vi "quiz3.vi"() -> ()   [LabVIEW 2017]
panel:
  out "Tab Control":enum32{"Login", "Menu", "Add", "delete"}(tab)
  in  "Ingresar":bool
  in  "Contraseña":string
  in  "Usuario":string
  in  "Delete Button":bool
  in  "Add Button":bool
  in  "Home Button":bool
  out "Cusuario":string
  in  "Previous Button":bool
  in  "AddContraseña":string
  in  "AddUsuario":string
  in  "Agregar":bool
  out "Agregado":bool
  in  "Cancel Button":bool
  in  "DeleteUsuario 2":string
  in  "Previous Button 2":bool
  out "text":string
  # "USTED INGRESO CON EL USUARIO"
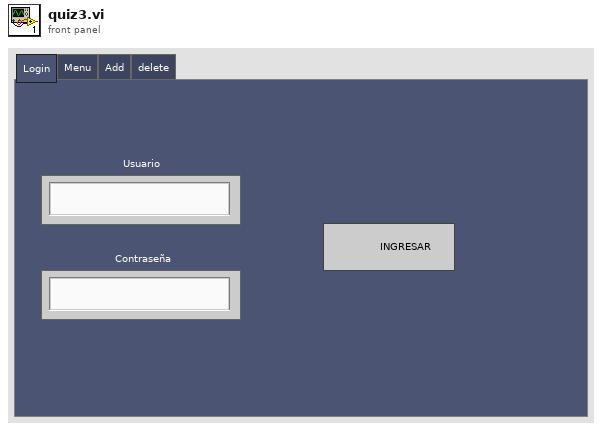
[diagram p1: front panel]
types:
  T1 = enum16{"open", "replace", "create", "open or create", "replace or create", "replace or create with confirmation"}
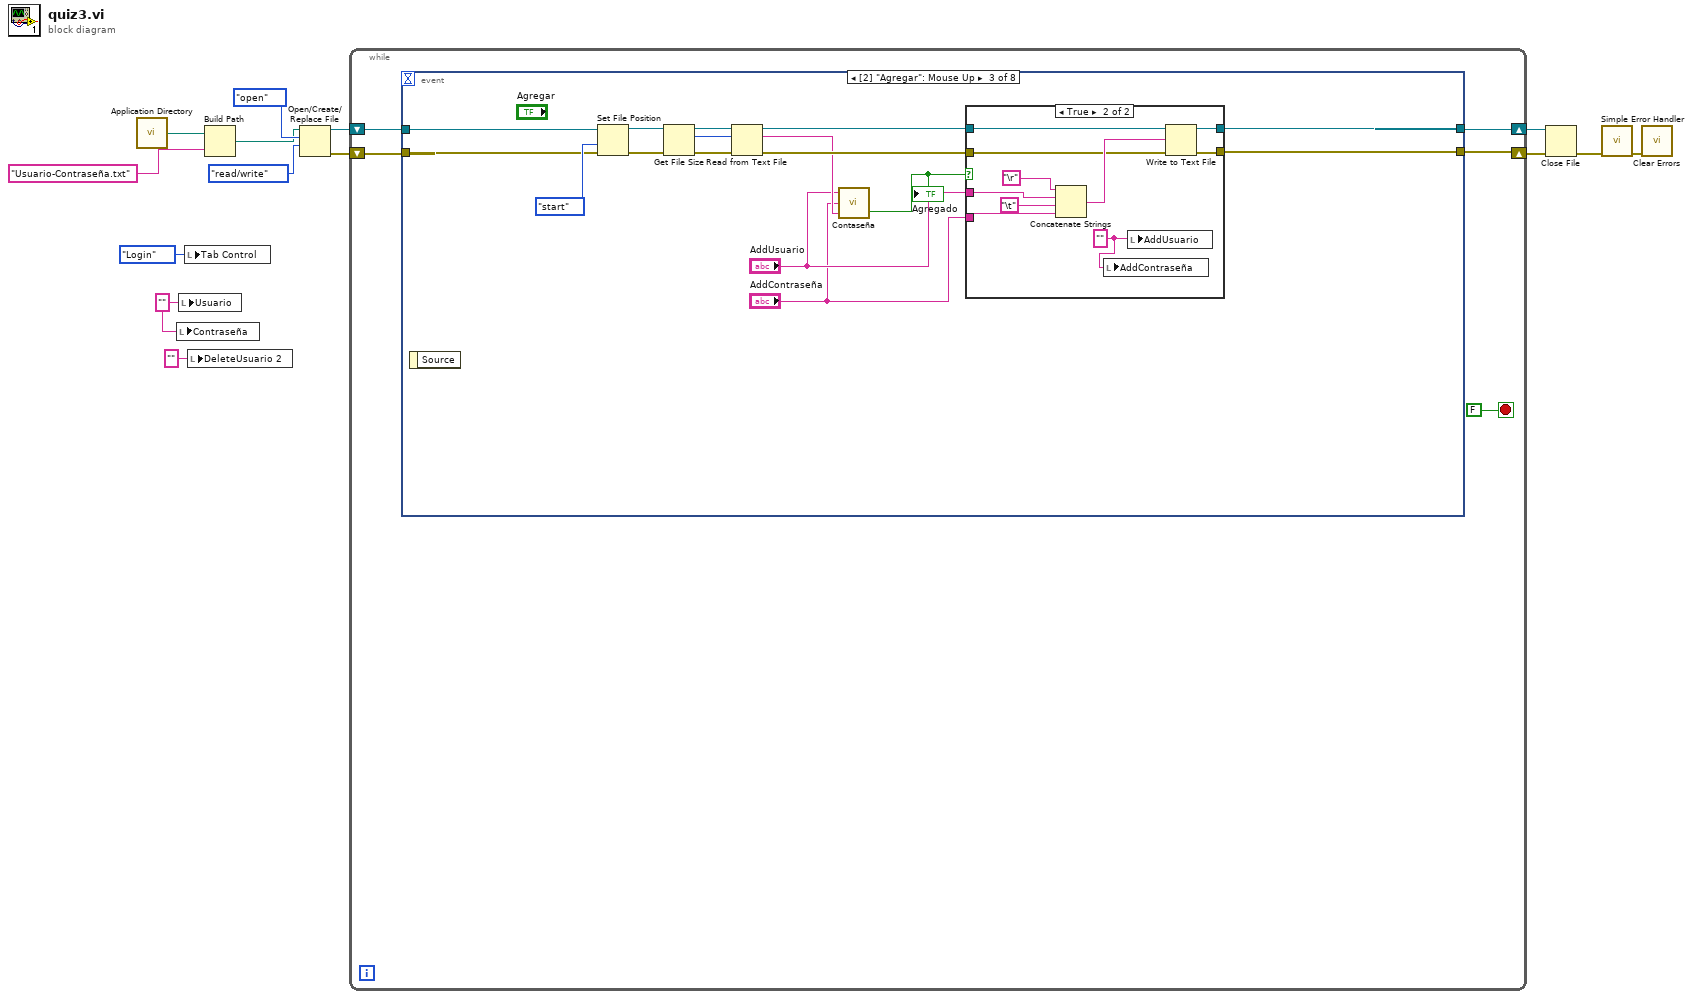
[diagram p0: block diagram]
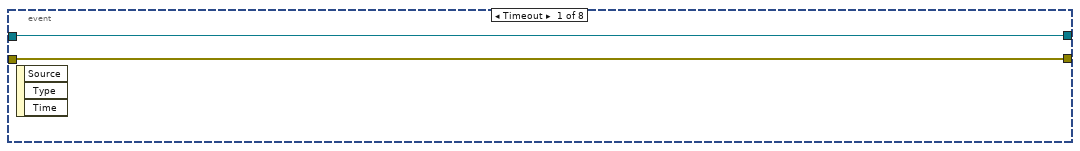
[diagram p2: hidden frame]
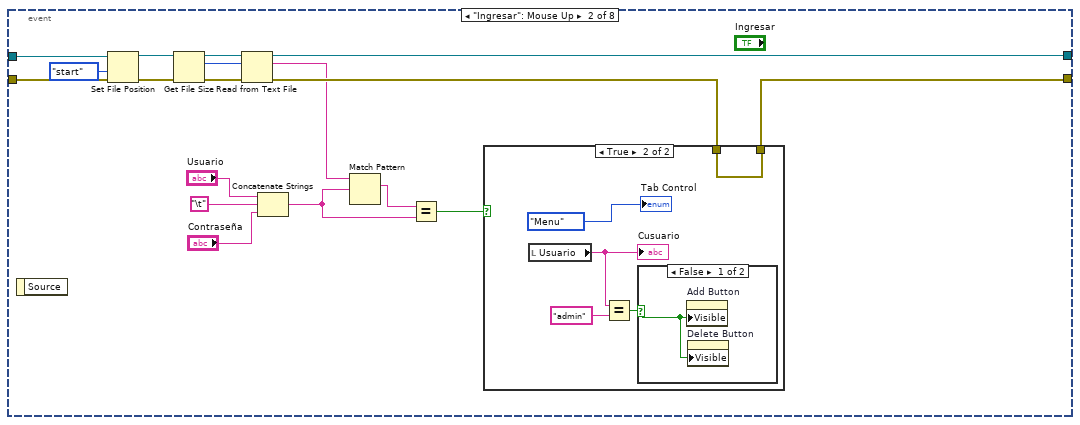
[diagram p3: hidden frame]
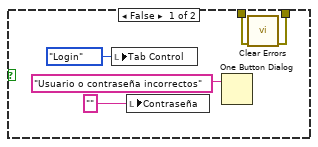
[diagram p4: hidden frame]
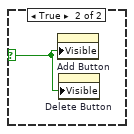
[diagram p5: hidden frame]
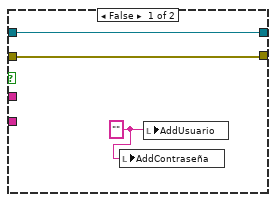
[diagram p6: hidden frame]
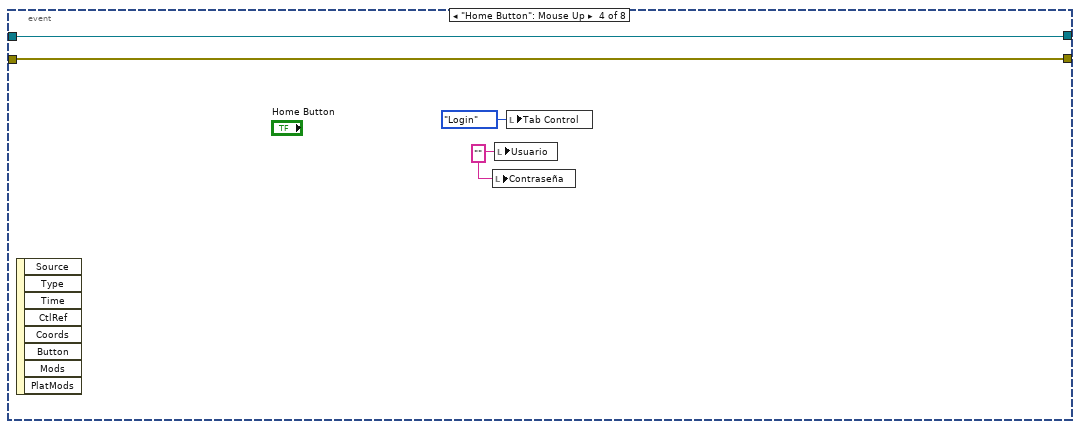
[diagram p7: hidden frame]
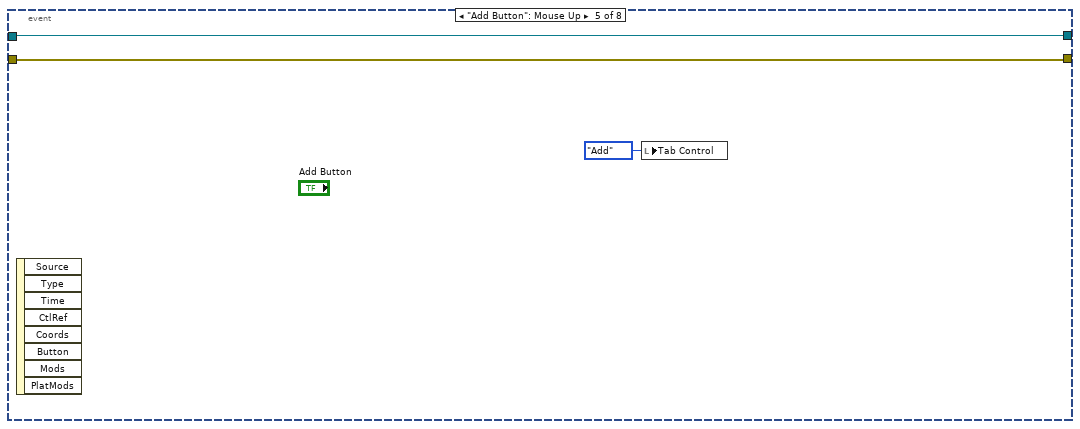
[diagram p8: hidden frame]
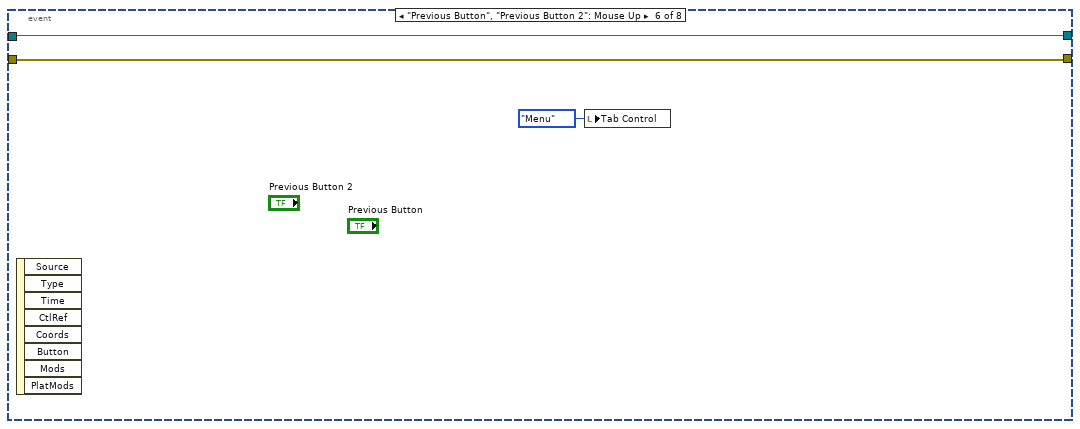
[diagram p9: hidden frame]
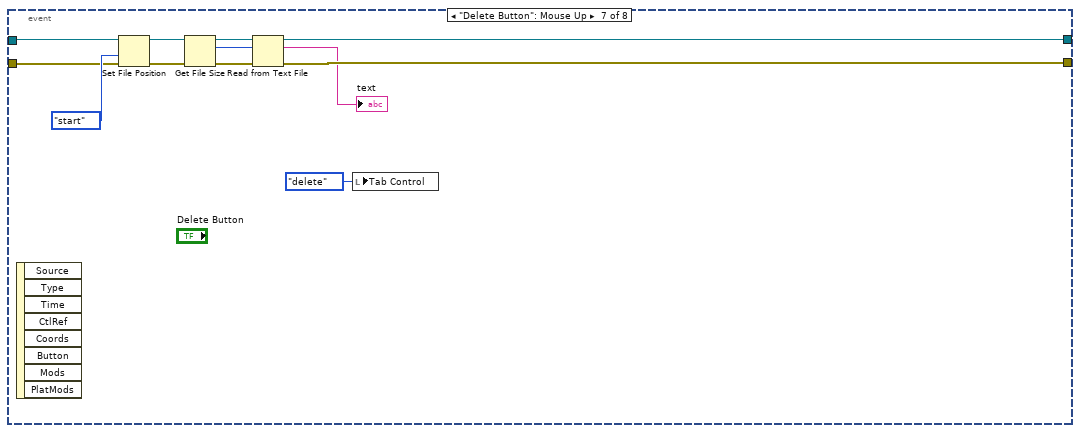
[diagram p10: hidden frame]
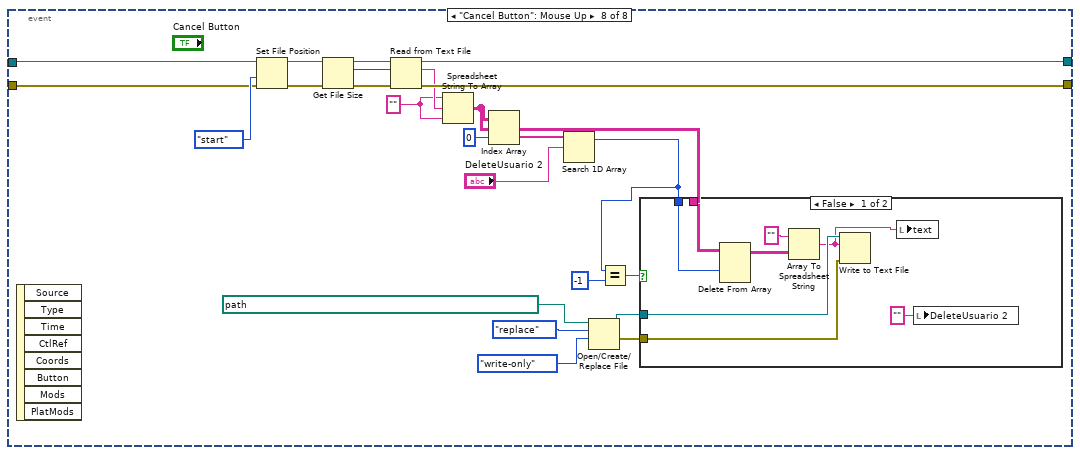
[diagram p11: hidden frame]
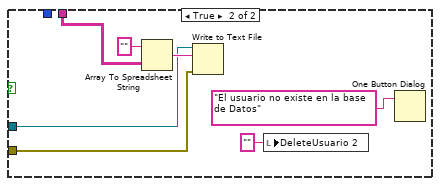
[diagram p12: hidden frame]
diagram:
  w5 = "" ("Usuario")
  n1 = call <vilib>:"Application Directory.vi"() -> ("Application Directory"=w14:path)
  n2 = local write "Contraseña"(w5) -> ()
  n3 = local write "Usuario"(w5) -> ()
  n4 = local write "Tab Control"(enum32{"Login", "Menu", "Add", "delete"}."Login" ("Tab Control")) -> ()
  n5 = local write "DeleteUsuario 2"("" ("DeleteUsuario 2")) -> ()
  n6 = Build Path(base path=w14, name or relative path="Usuario-Contraseña.txt") -> (appended path=w6:path)
  n7 = Open/Create/Replace File(file path (use dialog)=w6, operation (0:open)=T1."open", access (0:read/write)=enum16{"read/write", "read-only", "write-only"}."read/write") -> (refnum out=w2:refnum<file>, error out=w1:errorcluster)  [unwired: 3 in, 1 out]
  n8 = while {
    shift-right: [w16] -> w8
    shift-left: w2 -> [w17]
    shift-right: [w15] -> w7
    shift-left: w1 -> [w18]
    stop <- FALSE stop-if-true
    n9 = event shown="[2] \"Agregar\": Mouse Up" {
      selector: _ -> [_ _ _ _ _ _ _ _]
      dyn-events: _ -> [_ _ _ _ _ _ _ _]
      timeout: _ -> [_ _ _ _ _ _ _ _]
      tunnel: w18 -> [w20 w39 w55 w82 w86 w89 w93 w120]
      tunnel: [w21 w31 w67 w83 w87 w90 w94 w116] -> w16
      tunnel: [w20 w26 w66 w82 w86 w89 w92 w115] -> w15
      tunnel: w17 -> [w21 w28 w56 w83 w87 w90 w95 w119]
      event Timeout {
        n10 = event-data() -> ()  [unwired: 1 in, 3 out]
      }
      event "Ingresar": Mouse Up {
        n11 = event-data() -> ()  [unwired: 1 in, 1 out]
        n12 = Set File Position(refnum=w28, from (0:start)=enum16{"start", "end", "current"}."start", error in=w39) -> (refnum out=w37:refnum<file>, error out=w38:errorcluster)  [unwired: 1 in]
        n13 = Get File Size(file=w37, error in=w38) -> (refnum out=w24:refnum<file>, size (in bytes)=w36:i64, 0:w35:errorcluster)
        n14 = Read from Text File(file (use dialog)=w24, count=w36, error in=w35) -> (refnum out=w31:refnum<file>, text=w22:string, error out=w27:errorcluster)  [unwired: 1 in, 1 out]
        n15 = Concatenate Strings("Usuario", "\t", "Contraseña") -> (w29:string)
        n16 = Match Pattern(string=w22, regular expression=w29) -> (match substring=w30:string)  [unwired: 1 in, 3 out]
        n17 = Equal?(x=w30, y=w29) -> (x = y?=w33:bool)
        n18 = case shown="True" w33 {
          tunnel: [w42 w49] -> w26
          tunnel: w27 -> [w41 w49]
          frame False {
            n19 = local write "Tab Control"(enum32{"Login", "Menu", "Add", "delete"}."Login" ("Tab Control")) -> ()
            n20 = local write "Contraseña"("" ("Usuario")) -> ()
            n21 = One Button Dialog(message="Usuario o contraseña incorrectos") -> ()  [unwired: 1 in, 1 out]
            n22 = call <vilib>:"Clear Errors.vi"("error in (no error)"=w41) -> ("error out"=w42:errorcluster)  [unwired: 5 in, 1 out]
          }
          frame True {
            n23 = local read "Usuario"() -> (w47:string)
            "Cusuario" <- w47
            n24 = Equal?(x=w47, y="admin") -> (x = y?=w48:bool)
            n25 = case shown="False" w48 {
              selector: w48 -> [w50 w51]
              frame False {
                n26 = property on="Add Button" class="Bool (strict)"("Visible"=w50) -> ()  [unwired: 2 in, 2 out]
                n27 = property on="Delete Button" class="Bool (strict)"("Visible"=w50) -> ()  [unwired: 2 in, 2 out]
              }
              frame True {
                n28 = property on="Add Button" class="Bool (strict)"("Visible"=w51) -> ()  [unwired: 2 in, 2 out]
                n29 = property on="Delete Button" class="Bool (strict)"("Visible"=w51) -> ()  [unwired: 2 in, 2 out]
              }
            }
            "Tab Control" <- enum32{"Login", "Menu", "Add", "delete"}."Menu" ("Tab Control")
          }
        }
      }
      event "Agregar": Mouse Up {
        n30 = event-data() -> ()  [unwired: 1 in, 1 out]
        n31 = Set File Position(refnum=w56, from (0:start)=enum16{"start", "end", "current"}."start", error in=w55) -> (refnum out=w63:refnum<file>, error out=w64:errorcluster)  [unwired: 1 in]
        n32 = Get File Size(file=w63, error in=w64) -> (refnum out=w60:refnum<file>, size (in bytes)=w62:i64, 0:w61:errorcluster)
        n33 = Read from Text File(file (use dialog)=w60, count=w62, error in=w61) -> (refnum out=w58:refnum<file>, text=w54:string, error out=w57:errorcluster)  [unwired: 1 in, 1 out]
        n34 = call "Contaseña.vi"("spreadsheet string"=w54, "AddContraseña"="AddContraseña", "addUsuario"="AddUsuario") -> ("result"=w65:bool)  [unwired: 1 out]
        "Agregado" <- w65
        n35 = case shown="True" w65 {
          tunnel: [w70 w80] -> w67
          tunnel: [w69 w79] -> w66
          tunnel: w58 -> [w70 w75]
          tunnel: w57 -> [w69 w74]
          tunnel: "AddUsuario" -> [_ w73]
          tunnel: "AddContraseña" -> [_ w72]
          frame False {
            w68 = "" ("Usuario")
            n36 = local write "AddContraseña"(w68) -> ()
            n37 = local write "AddUsuario"(w68) -> ()
          }
          frame True {
            w71 = "" ("Usuario")
            n38 = Concatenate Strings("\r", w73, "\t", w72) -> (w78:string)
            n39 = local write "AddContraseña"(w71) -> ()
            n40 = local write "AddUsuario"(w71) -> ()
            n41 = Write to Text File(file (use dialog)=w75, text=w78, error in=w74) -> (refnum out=w80:refnum<file>, error out=w79:errorcluster)  [unwired: 1 in, 1 out]
          }
        }
      }
      event "Home Button": Mouse Up {
        w84 = "" ("Usuario")
        n42 = event-data() -> ()  [unwired: 1 in, 8 out]
        n43 = local write "Contraseña"(w84) -> ()
        n44 = local write "Usuario"(w84) -> ()
        n45 = local write "Tab Control"(enum32{"Login", "Menu", "Add", "delete"}."Login" ("Tab Control")) -> ()
      }
      event "Add Button": Mouse Up {
        n46 = event-data() -> ()  [unwired: 1 in, 8 out]
        n47 = local write "Tab Control"(enum32{"Login", "Menu", "Add", "delete"}."Add" ("Tab Control")) -> ()
      }
      event "Previous Button", "Previous Button 2": Mouse Up {
        n48 = event-data() -> ()  [unwired: 1 in, 8 out]
        n49 = local write "Tab Control"(enum32{"Login", "Menu", "Add", "delete"}."Menu" ("Tab Control")) -> ()
      }
      event "Delete Button": Mouse Up {
        n50 = event-data() -> ()  [unwired: 1 in, 8 out]
        n51 = Set File Position(refnum=w95, from (0:start)=enum16{"start", "end", "current"}."start", error in=w93) -> (refnum out=w100:refnum<file>, error out=w101:errorcluster)  [unwired: 1 in]
        n52 = Get File Size(file=w100, error in=w101) -> (refnum out=w97:refnum<file>, size (in bytes)=w99:i64, 0:w98:errorcluster)
        n53 = Read from Text File(file (use dialog)=w97, count=w99, error in=w98) -> (refnum out=w94:refnum<file>, text=→"text":string, error out=w92:errorcluster)  [unwired: 1 in, 1 out]
        n54 = local write "Tab Control"(enum32{"Login", "Menu", "Add", "delete"}."delete" ("Tab Control")) -> ()
      }
      event "Cancel Button": Mouse Up {
        w112 = "" ("format string")
        n55 = event-data() -> ()  [unwired: 1 in, 8 out]
        n56 = Set File Position(refnum=w119, from (0:start)=enum16{"start", "end", "current"}."start", error in=w120) -> (refnum out=w125:refnum<file>, error out=w126:errorcluster)  [unwired: 1 in]
        n57 = Get File Size(file=w125, error in=w126) -> (refnum out=w122:refnum<file>, size (in bytes)=w124:i64, 0:w123:errorcluster)
        n58 = Read from Text File(file (use dialog)=w122, count=w124, error in=w123) -> (refnum out=w116:refnum<file>, text=w113:string, error out=w115:errorcluster)  [unwired: 1 in, 1 out]
        n59 = Spreadsheet String To Array(format string=w112, spreadsheet string=w113, array type (2D Dbl)=w112) -> (array=w108:string[][])  [unwired: 1 in]
        n60 = Index Array(array=w108, index (col)=0 ("disabled index (col)")) -> (element=w110:string[])  [unwired: 1 in]
        n61 = Search 1D Array(1D array=w110, element="DeleteUsuario 2") -> (index of element=w104:i32)  [unwired: 1 in]
        n62 = Open/Create/Replace File(file path (use dialog)=path "D:/2019-1/Programacion 2/quiz 3/Usuario-Contraseña.txt", operation (0:open)=T1."replace", access (0:read/write)=enum16{"read/write", "read-only", "write-only"}."write-only") -> (refnum out=w107:refnum<file>, error out=w106:errorcluster)  [unwired: 3 in, 1 out]
        n63 = Equal?(x=w104, y=-1) -> (x = y?=w105:bool)
        n64 = case shown="False" w105 {
          tunnel: w108 -> [w134 w137]
          tunnel: w104 -> [w133 _]
          tunnel: w107 -> [w131 w136]
          tunnel: w106 -> [w130 w135]
          frame False {
            n65 = Delete From Array(array=w134, index (row)=w133) -> (array with subset deleted=w132:string[][])  [unwired: 2 in, 1 out]
            n66 = Array To Spreadsheet String(array=w132, 3:"" ("format string")) -> (spreadsheet string=w128:string)  [unwired: 1 in]
            n67 = Write to Text File(file (use dialog)=w131, text=w128, error in=w130) -> ()  [unwired: 1 in, 3 out]
            n68 = local write "text"(w128) -> ()
            n69 = local write "DeleteUsuario 2"("" ("DeleteUsuario 2")) -> ()
          }
          frame True {
            n70 = Array To Spreadsheet String(array=w137, 3:"" ("format string")) -> (spreadsheet string=w139:string)  [unwired: 1 in]
            n71 = Write to Text File(file (use dialog)=w136, text=w139, error in=w135) -> ()  [unwired: 1 in, 3 out]
            n72 = local write "DeleteUsuario 2"("" ("DeleteUsuario 2")) -> ()
            n73 = One Button Dialog(message="El usuario no existe en la base de Datos") -> ()  [unwired: 1 in, 1 out]
          }
        }
      }
    }
  }
  n74 = Close File(refnum=w8, error in=w7) -> (error out=w9:errorcluster)  [unwired: 1 out]
  n75 = call <vilib>:"Simple Error Handler.vi"("error in (no error)"=w9) -> ("error out"=w10:errorcluster)  [unwired: 4 in, 4 out]
  n76 = call <vilib>:"Clear Errors.vi"("error in (no error)"=w10) -> ()  [unwired: 5 in, 2 out]
